vi "UTF8 LV80.vi"(1 "utf-8 text":string) -> (0 "text out":string)   [LabVIEW 2020]
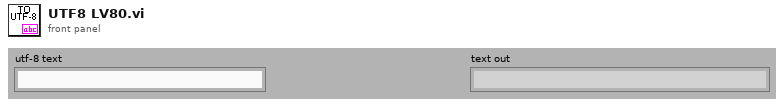
[diagram p1: front panel]
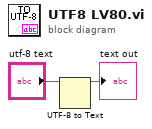
[diagram p0: block diagram]
diagram:
  n1 = UTF-8 to Text(11:"utf-8 text") -> (3:→"text out":string)  [unwired: 2 in, 1 out]
